vi "AI_ReadRawData16.vi"(0 "Task ID":u32, 2 "count":i32, 3 "error in (no error)":errorcluster) -> (7 "Task ID":u32, 8 "data":u16[](array[numeric]), 9 "error out":errorcluster)   [LabVIEW 2015]
uses:
  Windows/System32/AdvLvDaq.dll
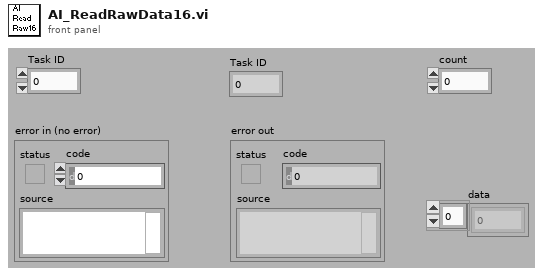
[diagram p1: front panel]
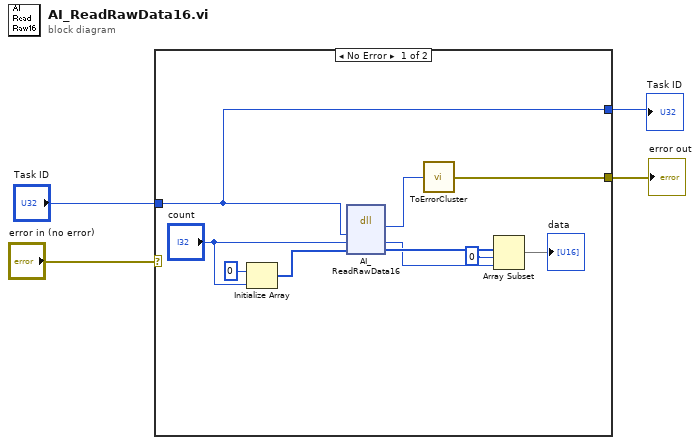
[diagram p0: block diagram]
diagram:
  n1 = case shown="No Error" "error in (no error)" {
    selector: "error in (no error)" -> [_ w15]
    tunnel: "Task ID" -> [w12 w16]
    tunnel: [w13 w15] -> w2
    tunnel: [w12 w16] -> w1
    frame No Error {
      n2 = Initialize Array(u16 0 ("element"), "count") -> (w11:u16[])
      n3 = dll-call lib="C:/Windows/System32/AdvLvDaq.dll" fn="AI_ReadRawData16"("taskId"=w12, "count"="count", "data"=w11) -> ("return type"=w14:i32, "count"=w8:i32, "data"=w9:u16[])  [unwired: 4 in, 2 out]
      n4 = call "ToErrorCluster.vi"("error code"=w14) -> ("error out"=w13:errorcluster)
      n5 = Array Subset(array=w9, index=0, length=w8) -> (→"data":u16[])
    }
    frame Error {
    }
  }
  "error out" <- w2
  "Task ID" <- w1
